vi "AFG_Waveform_settings.vi"(0 "amplitude (1)":dbl=1.0, 1 "frequency (1000000)":dbl=100.0, 2 "instrument handle":refnum<k15>="USB0::0x0699::0x0340::C012041::INSTR") -> ()   [LabVIEW 2015]
panel:
  out "error out":errorcluster {"code" format="%.0x"}
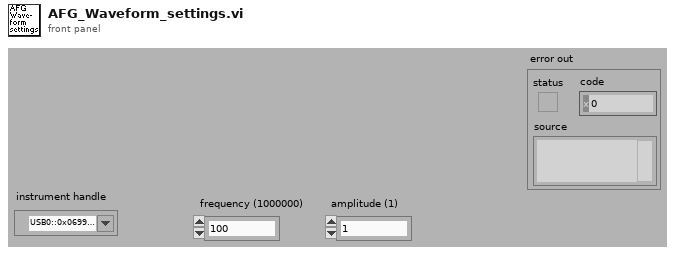
[diagram p1: front panel]
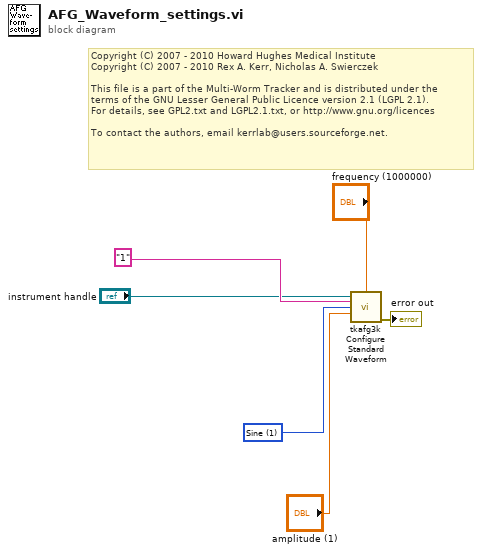
[diagram p0: block diagram]
diagram:
  w5 = 1 items=["Sine"=1, "Square"=2, "Pulse"=1002, "Ramp"=1001, "Noise"=1003, "DC"=6, "Sin(x)/x"=1004, "Gaussian"=1005, "Lorentz"=1006, "Exponential Rise"=1007, "Exponential Decay"=1008, "Haversine"=1009] ("waveform (Sine)")
  # "Copyright (C) 2007 - 2010 Howard Hughes Medical Institute\nCopyright (C) 2007 - 2010 Rex A. Kerr, Nicholas A. Swierczek\n \nThis file is a part of the Multi-Worm Tracker and is distributed under the\nterms of the GNU Lesser General Public Licence version 2.1 (LGPL 2.1).\nFor details, see GPL2.txt and LGPL2.1.txt, or http://www.gnu.org/licences\n \nTo contact the authors, email kerrlab@users.sourceforge.net."
  n1 = call <instrlib>:"tkafg3k Configure Standard Waveform.vi"("instrument handle"="instrument handle", "frequency (1000000)"="frequency (1000000)", "channel name (\"1\")"="1" ("channel name (\"1\")"), "waveform (1: Sine)"=w5, "amplitude (1)"="amplitude (1)") -> ("error out"=→"error out":errorcluster)  [unwired: 9 in, 1 out]
